vi "Write Diagrams.vi"(5 "Diagrams":refnum<class "Diagram.lvclass">[](array[class]), 9 "Structure in":refnum<class "Structure.lvclass">) -> (3 "Structure out":refnum<class "Structure.lvclass">)   [LabVIEW 2014, in "Structure.lvclass"]
uses:
  Structure.lvclass
  Diagram/Diagram.lvclass
  Structure.lvclass/Structure.ctl
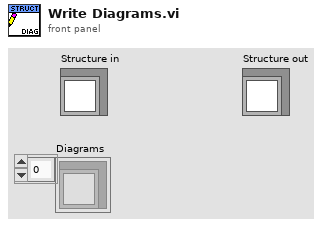
[diagram p1: front panel]
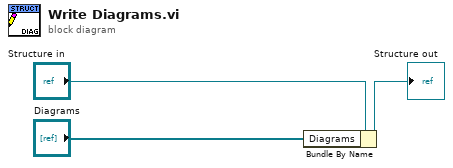
[diagram p0: block diagram]
diagram:
  n1 = Bundle By Name(cluster="Structure in", "Diagrams"="Diagrams") -> (→"Structure out":refnum<class "Structure.lvclass">)
